vi "Memory Throughput Test PXIe-796XR (Host).vi"() -> ()   [LabVIEW 2013]
doc: "This test writes to and reads from external memory at maximum data rates and reports the total measured throughput. Varying the write and read grant time will directly affect the memory efficiency. The larger the grant time, then the larger the througput, and the lower the grant time, then the lower the throughput \n\nDuring reads, the data is validated against an expected pattern. Failures will cause \"Read Data Error?\" to illuminate. To avoid read data errors, a full iteration of memory writes must be completed before starting the memory reads."
uses:
  <vilib>/FPGAPlugInAG/PXIe-7962R/niLvFpga_Open_PXIe-7962R.vi
  <vilib>/FPGAPlugInAG/PXIe-7962R/niLvFpga_Reset_PXIe-7962R.vi
  <vilib>/Utility/error.llb/Error Cluster From Error Code.vi
  <vilib>/rvi/errors/niLvFpgaAdjustHostInterfaceError.vi
  <vilib>/FPGAPlugInAG/PXIe-7962R/niLvFpga_Run_PXIe-7962R.vi
  <vilib>/FPGAPlugInAG/PXIe-7962R/niLvFpga_Close_PXIe-7962R.vi
  <vilib>/rvi/interface/nirviOpenFPGA/nirviOpenFPGA.xnode
  Program Files (x86)/National Instruments/LabVIEW 2013/examples/FlexRIO/External Memory/Memory Throughput Test/FPGA Bitfiles/MemoryThro_PXIe-7962R.lvbitx
  Program Files (x86)/National Instruments/LabVIEW 2013/examples/FlexRIO/External Memory/Memory Throughput Test/Memory Throughput Test PXIe-796XR (FPGA).vi
  <vilib>/rvi/interface/nirviMethod/nirviMethod.xnode
  <vilib>/rvi/interface/nirviReadWriteControl/nirviReadWriteControl.xnode
  <vilib>/rvi/interface/nirviCloseFPGA/nirviCloseFPGA.xnode
  NiFpgaLv.dll
panel:
  in  "Read Req Grant Time (Bank 1)":u16=1000 caption="Read Req Grant Time (clocks)"
  in  "Write Req Grant Time (Bank 1)":u16=1000 caption="Write Req Grant Time (clocks)"
  in  "Read Req Grant Time (Bank 0)":u16=1000 caption="Read Req Grant Time (clocks)"
  in  "Write Req Grant Time (Bank 0)":u16=1000 caption="Write Req Grant Time (clocks)"
  out "Read Data Error? (Bank 1)":bool caption="Read Data Error?"
  out "Read FIFO Overflow? (Bank 1)":bool caption="Read FIFO Overflow?"
  out "Read Data Error? (Bank 0)":bool caption="Read Data Error?"
  out "Read FIFO Overflow? (Bank 0)":bool caption="Read FIFO Overflow?"
  out "Current Read Data Lower (Bank 1)":u64 caption="Current Read Data Lower" format="%.0x"
  out "Read Throughput (bytes/sec) (Bank 1)":u32 caption="Read Throughput (bytes/sec)" format="%^.1e"
  out "Read Throughput (bytes/sec) (Bank 0)":u32 caption="Read Throughput (bytes/sec)" format="%^.1e"
  out "Current Read Data Lower (Bank 0)":u64 caption="Current Read Data Lower" format="%.0x"
  out "Current Read Address (Bank 1)":u32 caption="Current Read Address" format="%.0x"
  in  "Enable Reads? (Bank 1)":bool caption="Enable Reads?"
  in  "Enable Reads? (Bank 0)":bool caption="Enable Reads?"
  out "Current Read Address (Bank 0)":u32 caption="Current Read Address" format="%.0x"
  out "Current Write Data Lower (Bank 1)":u64 caption="Current Write Data Lower" format="%.0x"
  out "Current Write Address (Bank 1)":u32 caption="Current Write Address" format="%.0x"
  in  "Enable Writes? (Bank 1)":bool=TRUE caption="Enable Writes?"
  out "Write Throughput (bytes/sec) (Bank 1)":u32 caption="Write Throughput (bytes/sec)" format="%^.1e"
  in  "DRAM Size (elements) (Bank 1)":u32=16777216 caption="DRAM Size (elements)"
  out "Write Throughput (bytes/sec) (Bank 0)":u32 caption="Write Throughput (bytes/sec)" format="%^.1e"
  in  "Enable Writes? (Bank 0)":bool=TRUE caption="Enable Writes?"
  out "Current Write Data Lower (Bank 0)":u64 caption="Current Write Data Lower" format="%.0x"
  in  "DRAM Size (elements) (Bank 0)":u32=16777216 caption="DRAM Size (elements)"
  out "Current Write Address (Bank 0)":u32 caption="Current Write Address" format="%.0x"
  in  "stop":bool
  # "Bank 0"
  # "Bank 1"
  # "This test writes to and reads from external memory at maximum data rates and reports the total measured throughput.  Varying the write and read grant time will directly affect the memory efficiency.  The larger the grant time, then the larger the througput, and the lower the grant time, then the lower the throughput \n\nDuring reads, the data is validated against an expected pattern.  Failures will cause \"Read Data Error?\" to illuminate.  To avoid read data errors, a full iteration of memory writes must be completed before starting the memory reads."
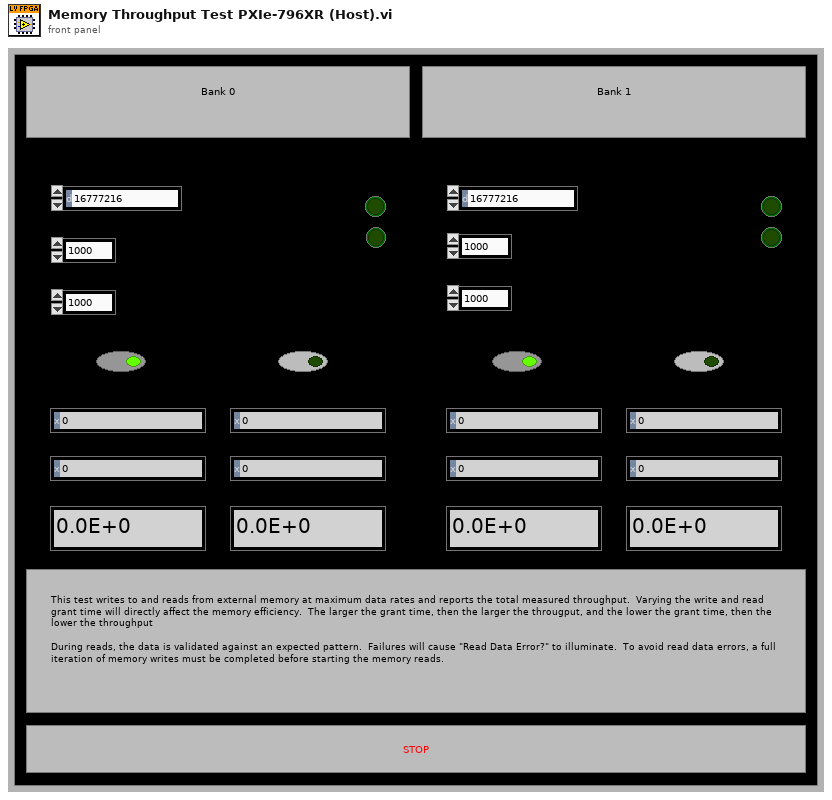
[diagram p1: front panel]
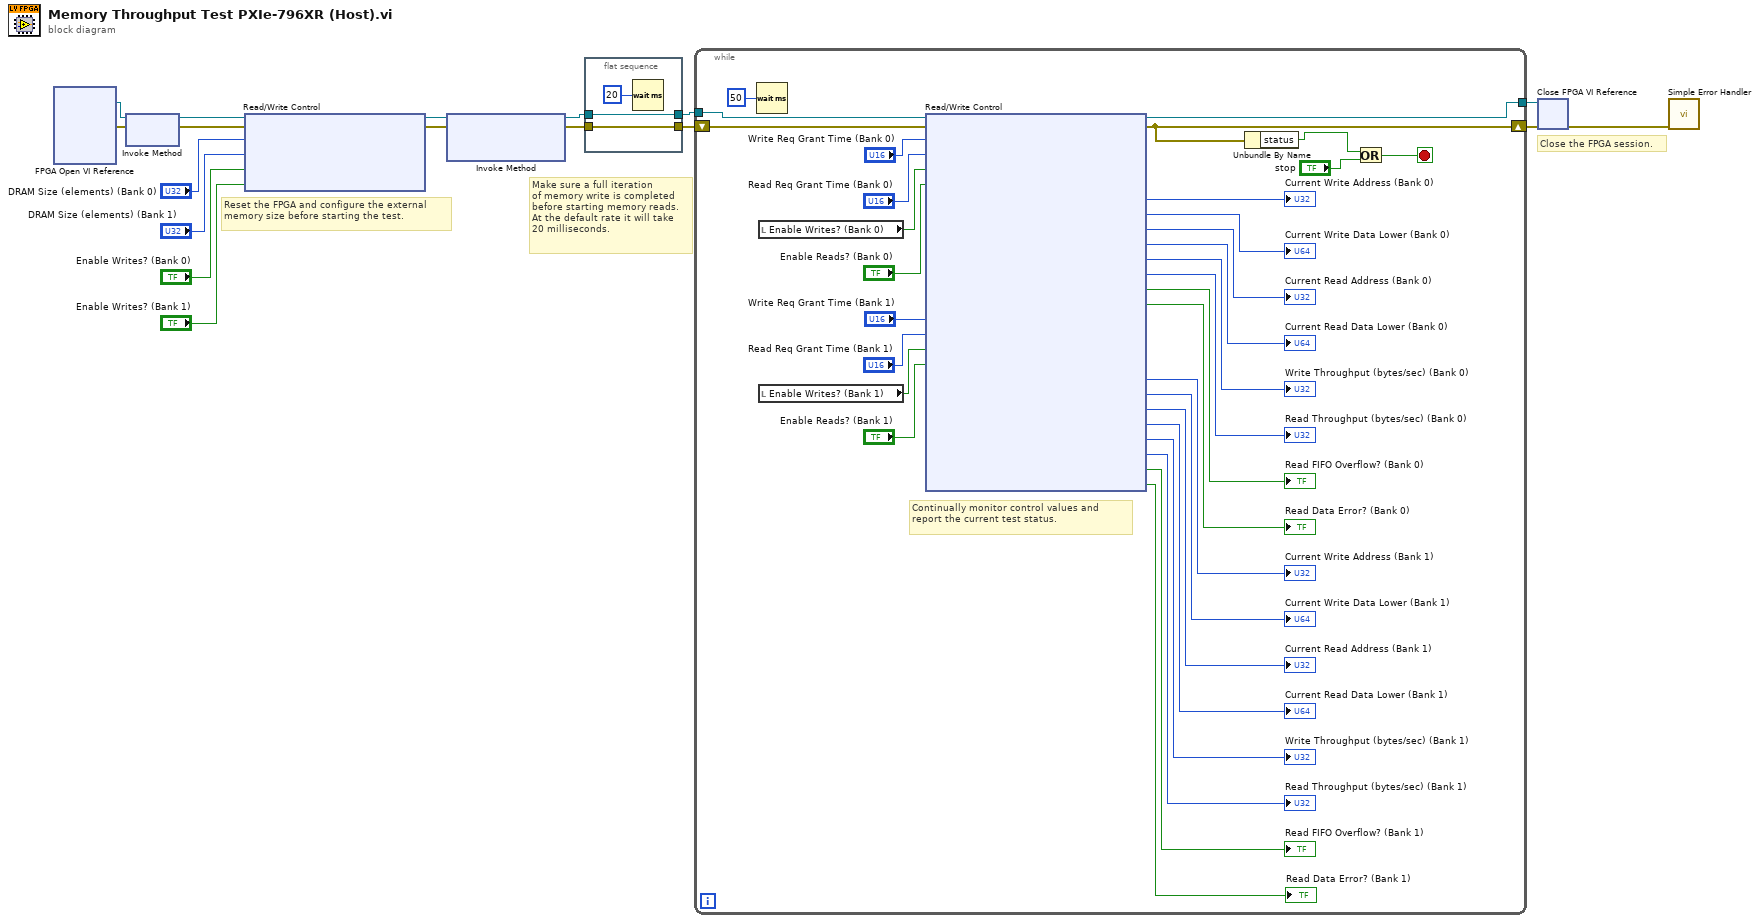
[diagram p0: block diagram]
diagram:
  # "Make sure a full iteration\nof memory write is completed\nbefore starting memory reads.\nAt the default rate it will take\n20 milliseconds."
  # "Close the FPGA session."
  # "Reset the FPGA and configure the external memory size before starting the test."
  n1 = xnode "FPGA Open VI Reference"() -> ("FPGA VI Reference Out"=w10:refnum<k20>, "error out"=w11:errorcluster)  [unwired: 2 in]
  n2 = xnode "Invoke Method"("FPGA VI Reference In"=w10, "error in"=w11) -> ("FPGA VI Reference Out"=w9:refnum<k20>, "error out"=w8:errorcluster)
  n3 = xnode "Read/Write Control"("FPGA VI Reference In"=w9, "error in"=w8, "DRAM Size (elements) (Bank 0)"="DRAM Size (elements) (Bank 0)", "DRAM Size (elements) (Bank 1)"="DRAM Size (elements) (Bank 1)", "Enable Writes? (Bank 0)"="Enable Writes? (Bank 0)", "Enable Writes? (Bank 1)"="Enable Writes? (Bank 1)") -> ("FPGA VI Reference Out"=w16:refnum<k20>, "error out"=w17:errorcluster)
  n4 = xnode "Invoke Method"("FPGA VI Reference In"=w16, "error in"=w17) -> ("FPGA VI Reference Out"=w4:refnum<k20>, "error out"=w3:errorcluster)  [unwired: 1 in]
  n5 = flat-sequence {
    tunnel: w4 -> [w20]
    tunnel: [w20] -> w6
    tunnel: w3 -> [w19]
    tunnel: [w19] -> w5
    frame #0 {
      n6 = Wait (ms)(milliseconds to wait=u32 20) -> ()  [unwired: 1 out]
    }
  }
  n7 = while {
    shift-right: [w47] -> w15
    shift-left: w5 -> [w45]
    tunnel: w6 -> [w46]
    tunnel: [w48] -> w7
    stop <- w52 stop-if-true
    # "Continually monitor control values and report the current test status."
    n8 = Wait (ms)(milliseconds to wait=u32 50) -> ()  [unwired: 1 out]
    n9 = local read "Enable Writes? (Bank 0)"() -> (w44:bool)
    n10 = local read "Enable Writes? (Bank 1)"() -> (w42:bool)
    n11 = xnode "Read/Write Control"("FPGA VI Reference In"=w46, "error in"=w45, "Write Req Grant Time (Bank 0)"="Write Req Grant Time (Bank 0)", "Read Req Grant Time (Bank 0)"="Read Req Grant Time (Bank 0)", "Enable Writes? (Bank 0)"=w44, "Enable Reads? (Bank 0)"="Enable Reads? (Bank 0)", "Write Req Grant Time (Bank 1)"="Write Req Grant Time (Bank 1)", "Read Req Grant Time (Bank 1)"="Read Req Grant Time (Bank 1)", "Enable Writes? (Bank 1)"=w42, "Enable Reads? (Bank 1)"="Enable Reads? (Bank 1)") -> ("FPGA VI Reference Out"=w48:refnum<k20>, "error out"=w47:errorcluster, "Current Write Address (Bank 0)"=→"Current Write Address (Bank 0)":u32, "Current Write Data Lower (Bank 0)"=→"Current Write Data Lower (Bank 0)":u64, "Current Read Address (Bank 0)"=→"Current Read Address (Bank 0)":u32, "Current Read Data Lower (Bank 0)"=→"Current Read Data Lower (Bank 0)":u64, "Write Throughput (bytes/sec) (Bank 0)"=→"Write Throughput (bytes/sec) (Bank 0)":u32, "Read Throughput (bytes/sec) (Bank 0)"=→"Read Throughput (bytes/sec) (Bank 0)":u32, "Read FIFO Overflow? (Bank 0)"=→"Read FIFO Overflow? (Bank 0)":bool, "Read Data Error? (Bank 0)"=→"Read Data Error? (Bank 0)":bool, "Current Write Address (Bank 1)"=→"Current Write Address (Bank 1)":u32, "Current Write Data Lower (Bank 1)"=→"Current Write Data Lower (Bank 1)":u64, "Current Read Address (Bank 1)"=→"Current Read Address (Bank 1)":u32, "Current Read Data Lower (Bank 1)"=→"Current Read Data Lower (Bank 1)":u64, "Write Throughput (bytes/sec) (Bank 1)"=→"Write Throughput (bytes/sec) (Bank 1)":u32, "Read Throughput (bytes/sec) (Bank 1)"=→"Read Throughput (bytes/sec) (Bank 1)":u32, "Read FIFO Overflow? (Bank 1)"=→"Read FIFO Overflow? (Bank 1)":bool, "Read Data Error? (Bank 1)"=→"Read Data Error? (Bank 1)":bool)
    n12 = Unbundle By Name(w47) -> ("status"=w50:bool)
    n13 = Or(x=w50, y="stop") -> (x .or. y?=w52:bool)
  }
  n14 = xnode "Close FPGA VI Reference"("FPGA VI Reference In"=w7, "error in"=w15) -> ("error out"=w14:errorcluster)
  n15 = call <vilib>:"Simple Error Handler.vi"("error in (no error)"=w14) -> ()  [unwired: 1 in, 8 out]
